vi "PreIni.vi"(8 "error in (no error)":errorcluster caption="错误输入（无错误）", 11 "zsActor输入":refnum<class "ActorWrapper.lvclass">) -> (0 "error out":errorcluster caption="错误输出", 3 "zsActor输出":refnum<class "ActorWrapper.lvclass">)   [LabVIEW 2014]
uses:
  zsActor/ActorWrapper.lvclass
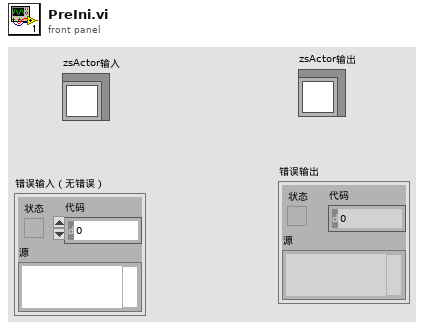
[diagram p1: front panel]
types:
  T1 = enum16{"OpenSlaveActor", "Idle", "StopSlaveActor"}
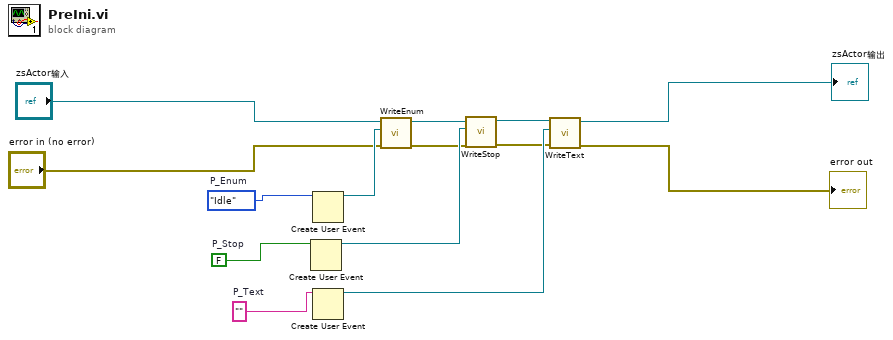
[diagram p0: block diagram]
diagram:
  w12 = ""  # P_Text
  w11 = FALSE  # P_Stop
  w10 = T1."Idle"  # P_Enum
  n1 = Create User Event(user event datatype=w11) -> (user event=w8:refnum<user-event>)  [unwired: 1 in, 1 out]
  n2 = Create User Event(user event datatype=w10) -> (user event=w9:refnum<user-event>)  [unwired: 1 in, 1 out]
  n3 = Create User Event(user event datatype=w12) -> (user event=w7:refnum<user-event>)  [unwired: 1 in, 1 out]
  n4 = call-dynamic "WriteEnum.vi"("error in (no error)"="error in (no error)", "Enum"=w9, "zsActor输入"="zsActor输入") -> ("error out"=w6:errorcluster, "zsActor输出"=w14:refnum<class "ActorWrapper.lvclass">)  [unwired: 7 in]
  n5 = call-dynamic "WriteStop.vi"("error in (no error)"=w6, "Stop"=w8, "zsActor输入"=w14) -> ("error out"=w5:errorcluster, "zsActor输出"=w13:refnum<class "ActorWrapper.lvclass">)  [unwired: 7 in]
  n6 = call-dynamic "WriteText.vi"("error in (no error)"=w5, "Text"=w7, "zsActor输入"=w13) -> ("error out"=→"error out":errorcluster, "zsActor输出"=→"zsActor输出":refnum<class "ActorWrapper.lvclass">)  [unwired: 7 in]
